vi "Shooter Simulator Globals.vi"() -> ()   [LabVIEW 2015]
uses:
  Shooter Simulator Sensor Data.ctl
panel:
  in  "R Shooter Power":dbl
  in  "L Shooter Power":dbl
  in  "Angle Motor Power":dbl
  in  "Sim Data":T1
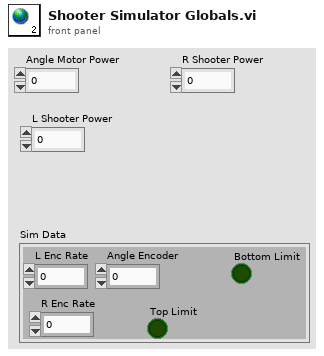
[diagram p1: front panel]
types:
  T1 = typedef "Shooter Simulator Sensor Data.ctl" = cluster{"L Enc Rate":dbl, "R Enc Rate":dbl, "Angle Encoder":dbl, "Top Limit":bool, "Bottom Limit":bool}
diagram:
